vi "final gps for recursive.vi"() -> ()   [LabVIEW 2014]
uses:
  <vilib>/FPGAPlugInAG/cRIO-9063/niLvFpga_Open_cRIO-9063.vi
  <vilib>/rvi/interface/common/dynamic/niFpgaDynamicAddResources.vi
  <vilib>/Utility/error.llb/Error Cluster From Error Code.vi
  <vilib>/rvi/errors/niLvFpgaAdjustHostInterfaceError.vi
  <vilib>/FPGAPlugInAG/Dynamic/niLvFpga_Close_Dynamic.vi
  <vilib>/rvi/interface/nirviOpenFPGA/nirviOpenFPGA.xnode
  akhil3/FPGA Bitfiles/trailswithgps_FPGATarget_recursiveakhil_QexfQQGvF84.lvbitx
  recursive akhil.vi
  <vilib>/rvi/interface/nirviReadWriteControl/nirviReadWriteControl.xnode
  <vilib>/rvi/interface/nirviCloseFPGA/nirviCloseFPGA.xnode
  NiFpgaLv.dll
  <vilib>/rvi/interface/Simulation/niFpgaSimulationCallBeginRW.vi
panel:
  out "LabVIEW time":timestamp
  out "GPS status":T1(ring)
  out "FPGA Timekeeper locked":bool
  out "offset from time reference":i32
  out "satellites available":u8
  out "UTC offset":i8
  out "UTC offset valid":bool
  out "voltage frequency":fxp<+/-,35,18>
  out "current frequency":fxp<+/-,35,18>
  out "Raw PPS Timestamp (TAI ns)":u64
  out "PPS TAI Timestamp":timestamp format="%<%.9X\n%x>T"
  out "PPS UTC Timestamp":timestamp format="%<%.9X\n%x>T"
  out "antenna status":T2(ring)
  out "Latitude (°)":fxp<+/-,28,8>
  out "Longitude (°)":fxp<+/-,29,9>
  out "Altitude (m)":fxp<+/-,24,17>
  out "rate of chage of frequency":fxp<+/-,17,17>
  out "Theta":fxp<+/-,22,10>[](array[numeric])
  out "Magnitude":fxp<+,60,17>[](array[numeric])
  out "element":fxp<+,60,17>
  out "array of clusters":T3(array[cluster])
  out "Current Phasors":picture
  in  "polar attributes 6":T4={"maximum"=0.0, "minimum"=0.0, "clip to min"=FALSE, "log?(F)"=FALSE, "grid color"=6710886, "plot color"=65280, "fmt and prec"={"format"=enum."Decimal", "precision"=0}, "visible section"=8} {"minimum" format="%0.2f"; "maximum" format="%0.2f"}
  out "element 2":fxp<+,60,17>
  out "array of clusters 2":T3(array[cluster])
  out "Voltage Phasors":picture
  in  "polar attributes 7":T4={"maximum"=0.0, "minimum"=0.0, "clip to min"=FALSE, "log?(F)"=FALSE, "grid color"=6710886, "plot color"=65280, "fmt and prec"={"format"=enum."Decimal", "precision"=0}, "visible section"=8} {"minimum" format="%0.2f"; "maximum" format="%0.2f"}
  out "GPS TIME":timestamp[](array[timestamp])
  in  "Numeric":i32
  out "frequency":fxp<+/-,35,18>[](array[numeric])
  out "ROCOF":fxp<+/-,17,17>[](array[numeric])
  out "Array":T5(array[cluster])
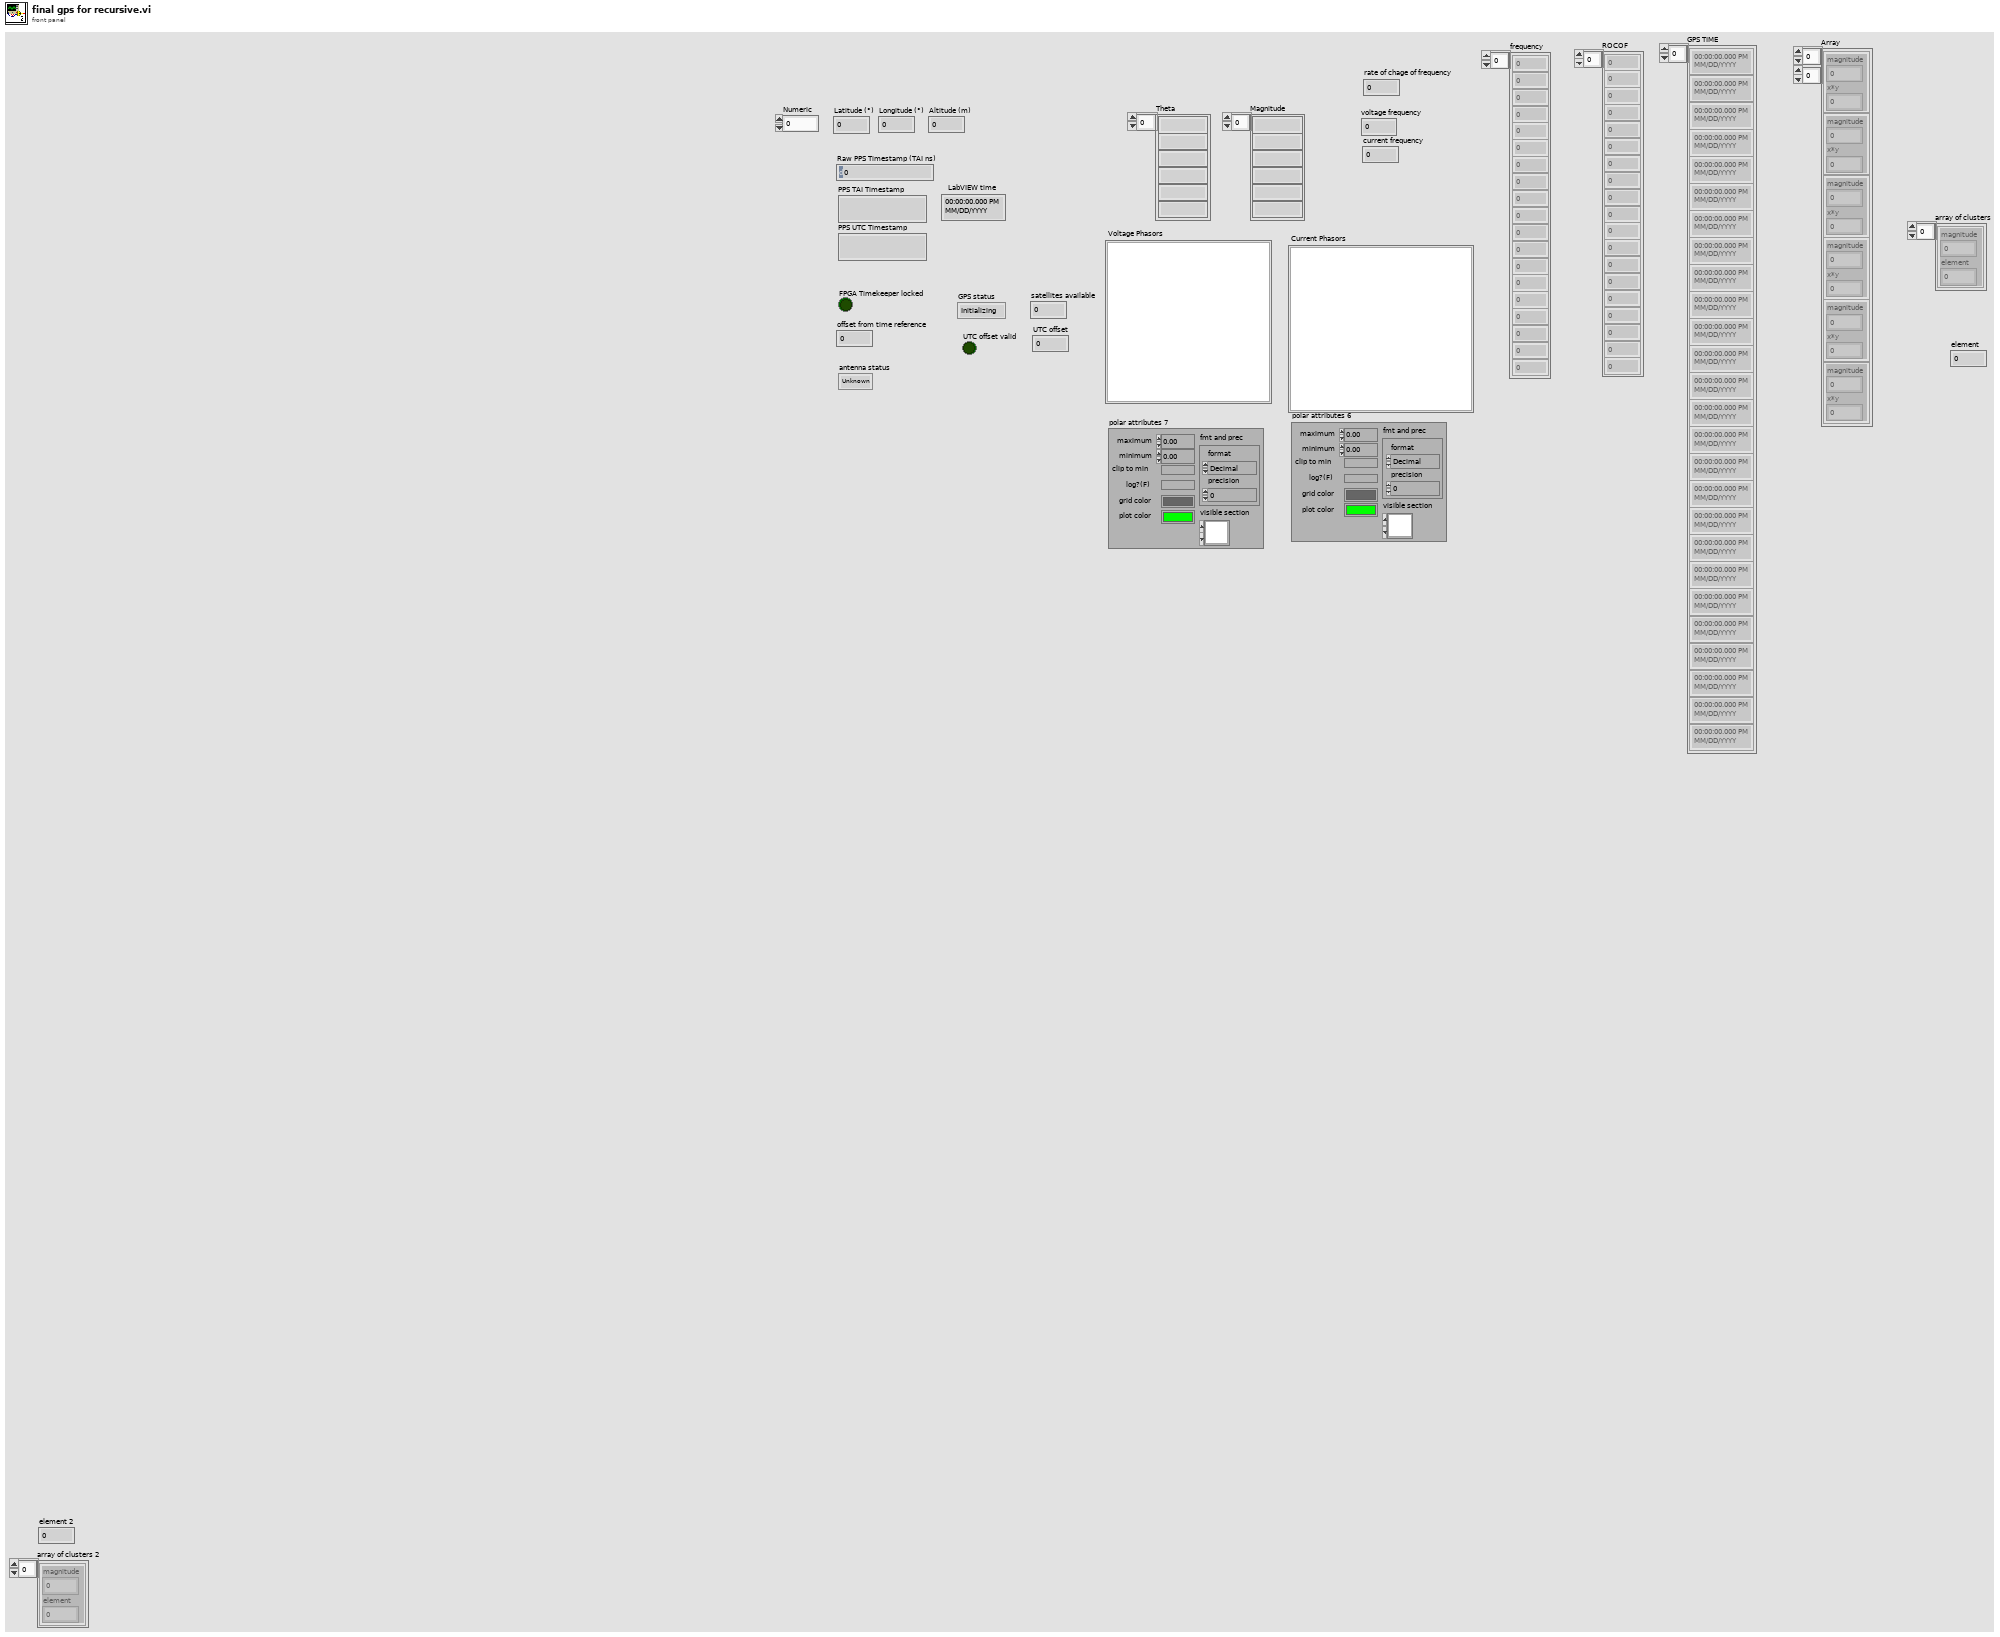
[diagram p1: front panel]
types:
  T1 = enum8{"Initializing", "Normal", "Unable to get fix"}
  T2 = enum8{"Unknown", "Normal", "Absent", "Overcurrent"}
  T3 = cluster{"magnitude":fxp<+,60,17>, "element":fxp<+/-,61,18>}[]
  T4 = cluster{"maximum":dbl, "minimum":dbl, "clip to min":bool, "log?(F)":bool, "grid color":u32, "plot color":u32, "fmt and prec":cluster{"format":enum8{"Decimal", "Scientific", "Engineering", "Binary", "Octal", "Hex"}, "precision":u8}, "visible section":u16}
  T5 = cluster{"magnitude":fxp<+,60,17>, "x*y":fxp<+/-,22,10>}[][]
  T6 = cluster{"magnitude":fxp<+,62,19>, "x*y":fxp<+/-,22,10>}[]
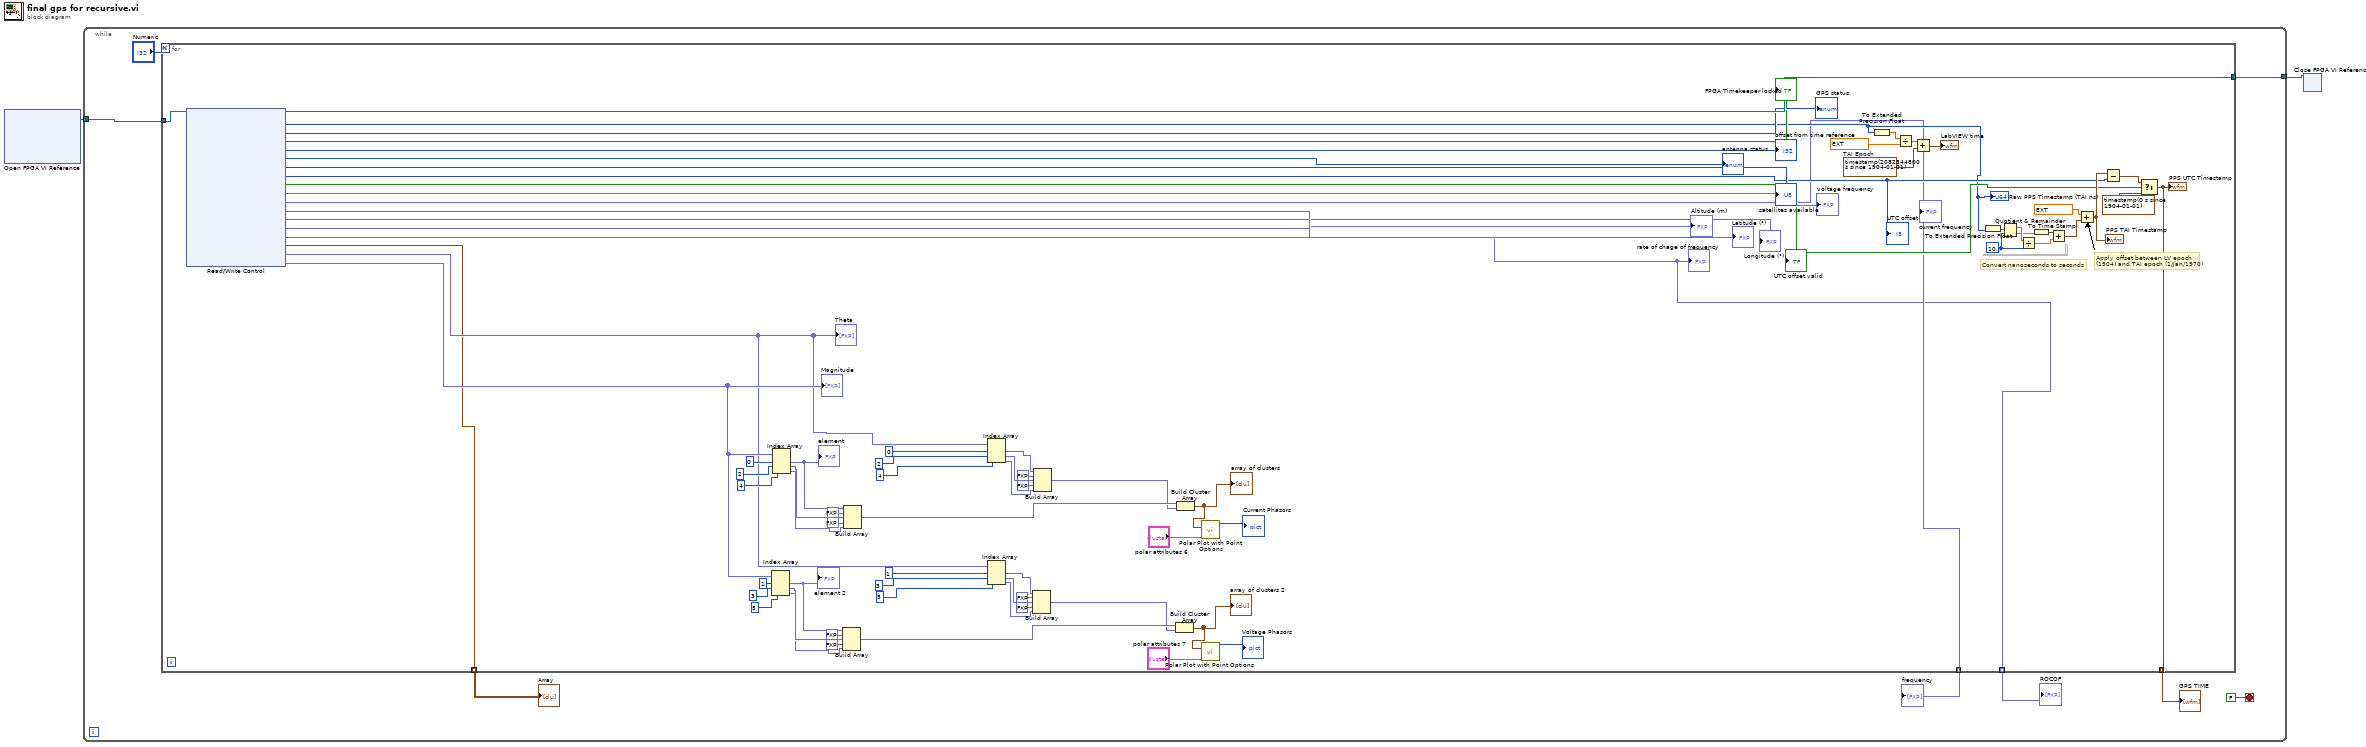
[diagram p0: block diagram]
diagram:
  n1 = xnode "Open FPGA VI Reference"() -> ("FPGA VI Reference Out"=w1:refnum<k20>)  [unwired: 2 in, 1 out]
  n2 = while {
    tunnel: [w9] -> w2
    tunnel: w1 -> [w7]
    stop <- FALSE stop-if-true
    n3 = for {
      N: "Numeric" -> [_]
      tunnel: w7 -> [w83]
      tunnel: [w82] -> w9
      tunnel: [w61] -> w10 mode=indexing
      tunnel: [w60] -> w5 mode=indexing
      tunnel: [w56] -> w4 mode=indexing
      tunnel: [w11] -> w3 mode=indexing
      w74 = u32 1000000000
      w86 = timestamp(2082844800 s since 1904-01-01)  # TAI Epoch
      # "Apply offset between LV epoch (1904) and TAI epoch (1/Jan/1970)"
      # "Convert nanoseconds to seconds"
      n4 = xnode "Read/Write Control"("FPGA VI Reference In"=w83) -> ("FPGA VI Reference Out"=w82:refnum<k20>, "FPGA Timekeeper time (ns) 2"=w62:u64, "GPS status"=→"GPS status":T1, "FPGA Timekeeper locked"=→"FPGA Timekeeper locked":bool, "offset from time reference"=→"offset from time reference":i32, "antenna status"=→"antenna status":T2, "satellites available"=→"satellites available":u8, "UTC offset"=w64:i8, "UTC offset valid"=w65:bool, "Voltage Frequency"=→"voltage frequency":fxp<+/-,35,18>, "current frequency"=w60:fxp<+/-,35,18>, "Latitude (°)"=→"Latitude (°)":fxp<+/-,28,8>, "Longitude (°)"=→"Longitude (°)":fxp<+/-,29,9>, "Altitude (m)"=→"Altitude (m)":fxp<+/-,24,17>, "ROCOF"=w56:fxp<+/-,17,17>, "Array"=w11:T6, "theta"=w12:fxp<+/-,22,10>[], "r"=w13:fxp<+,60,17>[])  [unwired: 1 in, 1 out]
      "UTC offset" <- w64
      "UTC offset valid" <- w65
      "current frequency" <- w60
      "Raw PPS Timestamp (TAI ns)" <- w62
      "rate of chage of frequency" <- w56
      "Theta" <- w12
      "Magnitude" <- w13
      n5 = Index Array(array=w13, index #1=1 ("index"), index #2=3 ("index"), index #3=5 ("index")) -> (element #1=w28:fxp<+,60,17>, element #2=w26:fxp<+,60,17>, element #3=w24:fxp<+,60,17>)
      "element 2" <- w28
      n6 = Index Array(array=w13, index #1=0 ("index"), index #2=2 ("index"), index #3=4 ("index")) -> (element #1=w49:fxp<+,60,17>, element #2=w47:fxp<+,60,17>, element #3=w45:fxp<+,60,17>)
      "element" <- w49
      n7 = Build Array(w28, fxp<+,60,17> 0.0 ("element"), w26, fxp<+,60,17> 0.0 ("element"), w24) -> (w18:fxp<+,60,17>[])
      n8 = Build Array(w49, fxp<+,60,17> 0.0 ("element"), w47, fxp<+,60,17> 0.0 ("element"), w45) -> (w39:fxp<+,60,17>[])
      n9 = Index Array(array=w12, index #1=1 ("index"), index #2=3 ("index"), index #3=5 ("index")) -> (element #1=w21:fxp<+/-,22,10>, element #2=w20:fxp<+/-,22,10>, element #3=w19:fxp<+/-,22,10>)
      n10 = Index Array(array=w12, index #1=0 ("index"), index #2=2 ("index"), index #3=4 ("index")) -> (element #1=w42:fxp<+/-,22,10>, element #2=w41:fxp<+/-,22,10>, element #3=w40:fxp<+/-,22,10>)
      n11 = Build Array(w21, fxp<+,60,17> 0.0 ("element"), w20, fxp<+,60,17> 0.0 ("element"), w19) -> (w17:fxp<+/-,61,18>[])
      n12 = Build Array(w42, fxp<+,60,17> 0.0 ("element"), w41, fxp<+,60,17> 0.0 ("element"), w40) -> (w38:fxp<+/-,61,18>[])
      n13 = Build Cluster Array(w18, w17) -> (w15:T3)
      "array of clusters 2" <- w15
      n14 = Build Cluster Array(w39, w38) -> (w36:T3)
      "array of clusters" <- w36
      n15 = call <vilib>:"Polar Plot with Point Options.vi"("data array [mag, phase (deg)]"=w15, "polar attributes"="polar attributes 7") -> ("new picture"=→"Voltage Phasors":picture)  [unwired: 13 in]
      n16 = call <vilib>:"Polar Plot with Point Options.vi"("data array [mag, phase (deg)]"=w36, "polar attributes"="polar attributes 6") -> ("new picture"=→"Current Phasors":picture)  [unwired: 13 in]
      n17 = To Extended Precision Float(1:w62) -> (0:w84:ext)
      n18 = Divide(x=w84, y=ext 1000000000.0) -> (x/y=w87:ext)
      n19 = Add(x=w87, y=w86) -> (x+y=→"LabVIEW time":timestamp)
      n20 = To Extended Precision Float(1:w62) -> (0:w76:ext)
      n21 = Quotient & Remainder(x=w76, y=w74) -> (x-y*floor(x/y)=w75:ext, floor(x/y)=w73:ext)
      n22 = Divide(x=w75, y=w74) -> (x/y=w71:ext)
      n23 = To Time Stamp(1:w73) -> (0:w72:timestamp)
      n24 = Add(x=w72, y=w71) -> (x+y=w70:timestamp)
      n25 = Add(x=ext 2082844800.0, y=w70) -> (x+y=w68:timestamp)
      "PPS TAI Timestamp" <- w68
      n26 = Subtract(x=w68, y=w64) -> (x-y=w67:timestamp)
      n27 = Select(t=w67, s=w65, f=timestamp(0 s since 1904-01-01)) -> (s? t:f=w61:timestamp)
      "PPS UTC Timestamp" <- w61
    }
    "GPS TIME" <- w10
    "frequency" <- w5
    "ROCOF" <- w4
    "Array" <- w3
  }
  n28 = xnode "Close FPGA VI Reference"("FPGA VI Reference In"=w2) -> ()  [unwired: 1 in, 1 out]
